vi "file -- get unique filename.vi"(10 "prefix":string="image", 11 "9w folder path":path=path "C:/data/RUS/Experiment/ProbeTest/Probe10/YBCO_6/sweep2/9w") -> (0 "appended path":path, 1 "name":string)   [LabVIEW 2017]
uses:
  <vilib>/regexp/Match Regular Expression.xnode
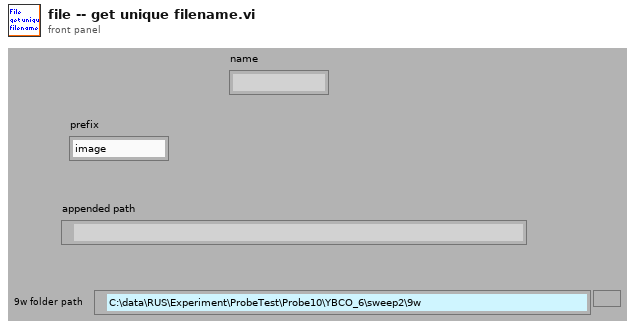
[diagram p1: front panel]
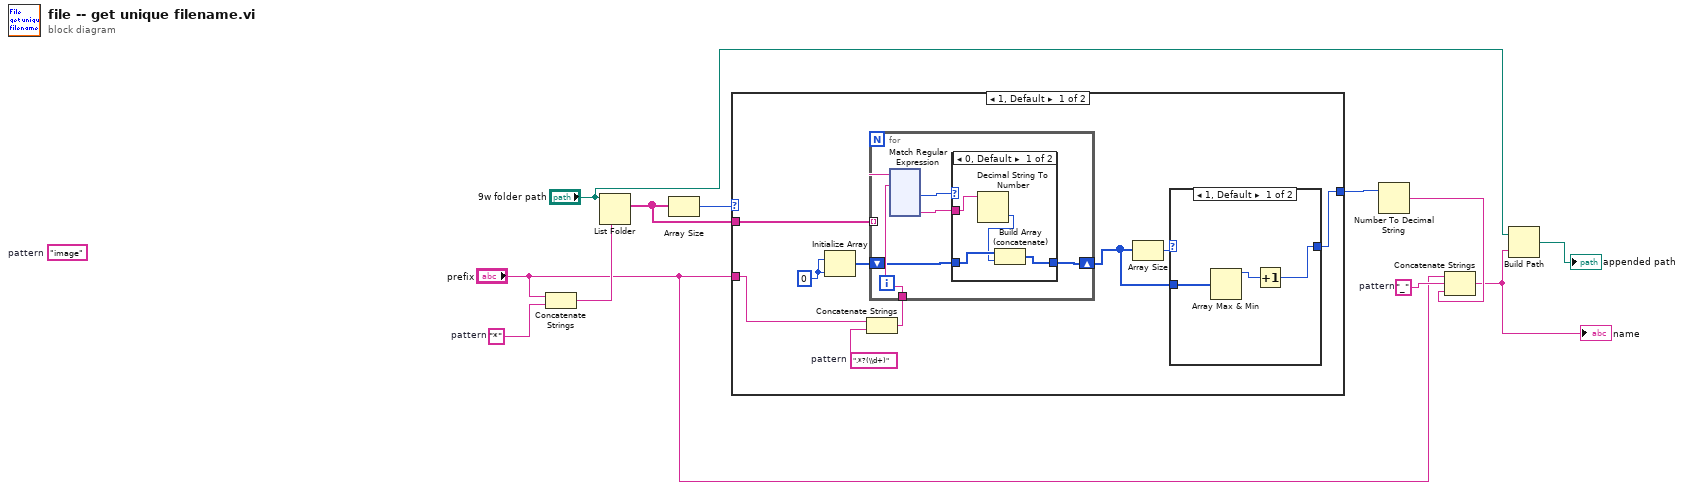
[diagram p0: block diagram]
diagram:
  w7 = "_"  # pattern
  w11 = "*"  # pattern
  (unwired) "image"  # pattern
  n1 = Concatenate Strings("prefix", w11) -> (w10:string)
  n2 = List Folder(path="9w folder path", pattern=w10) -> (filenames=w8:string[])  [unwired: 2 in, 3 out]
  n3 = Array Size(array=w8) -> (size(s)=w9:i32)
  n4 = case shown="1, Default" w9 {
    selector: w9 -> [_ w149]
    tunnel: "prefix" -> [w17 _]
    tunnel: w8 -> [w20 _]
    tunnel: [w13 w149] -> w5
    frame 1, Default {
      w15 = 0
      w19 = ".*?(\\d+)"  # pattern
      n5 = Initialize Array(w15, w15) -> (w16:i32[])
      n6 = Concatenate Strings(w17, w19) -> (w18:string)
      n7 = for {
        tunnel: w20 -> [w30] mode=indexing
        tunnel: w18 -> [w29]
        shift-right: [w27] -> w12
        shift-left: w16 -> [w26]
        n8 = xnode "Match Regular Expression"("input string"=w30, "regular expression"=w29) -> ("offset past match"=w28:i32, "submatch 1"=w25:string)  [unwired: 4 in, 4 out]
        n9 = case shown="0, Default" w28 {
          tunnel: [w33 w35] -> w27
          tunnel: w26 -> [w34 w35]
          tunnel: w25 -> [w32 _]
          frame 0, Default {
            n10 = Decimal String To Number(string=w32) -> (number=w31:i32)  [unwired: 2 in, 1 out]
            n11 = Build Array (concatenate)(w34, w31) -> (w33:i32[])
          }
          frame -1 {
          }
        }
      }
      n12 = Array Size(array=w12) -> (size(s)=w14:i32)
      n13 = case shown="1, Default" w14 {
        selector: w14 -> [_ w24]
        tunnel: [w21 w24] -> w13
        tunnel: w12 -> [w23 _]
        frame 1, Default {
          n14 = Array Max & Min(array=w23) -> (max value=w22:i32)  [unwired: 3 out]
          n15 = Increment(x=w22) -> (x+1=w21:i32)
        }
        frame 0 {
        }
      }
    }
    frame 0 {
    }
  }
  n16 = Number To Decimal String(number=w5) -> (decimal integer string=w6:string)  [unwired: 1 in]
  n17 = Concatenate Strings("prefix", w7, w6) -> (w4:string)
  "name" <- w4
  n18 = Build Path(base path="9w folder path", name or relative path=w4) -> (appended path=→"appended path":path)
